vi "PS (single).vi"(8 "error in (no error)":errorcluster, 11 "XY-data":cluster{"X-array":dbl[], "Y-array":dbl[]} {"Y-array" format="%.2p"; "X-array" format="%.2p"}) -> (0 "error out":errorcluster, 2 "Power Spectrum":cluster{"f0":dbl, "df":dbl, "magnitude":dbl[]} {"magnitude" format="%.2p"; "f0" format="%0.2p"; "df" format="%0.2p"}, 3 "XY-data out":cluster{"X-array":dbl[], "Y-array":dbl[]} {"Y-array" format="%.2p"; "X-array" format="%.2p"})   [LabVIEW 2019, in "xy_utilities.lvlib"]
doc: "Computes the Power Spectrum of <B>XY-data</B>. This VI is a wrapper for NI_MAPro.lvlib:FFT Power Spectrum and PSD.vi.\n\nWire data to the data input to determine the polymorphic instance to use or manually select the instance."
uses:
  xy_utilities.lvlib
  <vilib>/measure/NI_MAPro.lvlib
  <vilib>/measure/maspectr.llb/FFT Power Spectrum and PSD for 1 Chan.vi
  <vilib>/measure/maspectr.llb/Power Spectrum and PSD Export Mode.ctl
  <vilib>/measure/maresamp.llb/Resample Pair of Arrays (single shot).vi
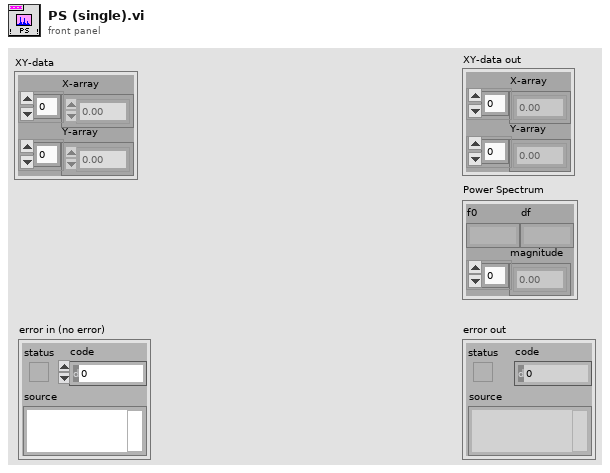
[diagram p1: front panel]
types:
  T1 = typedef "NI_MAPro.lvlib/Power Spectrum and PSD Export Mode.ctl" = u16
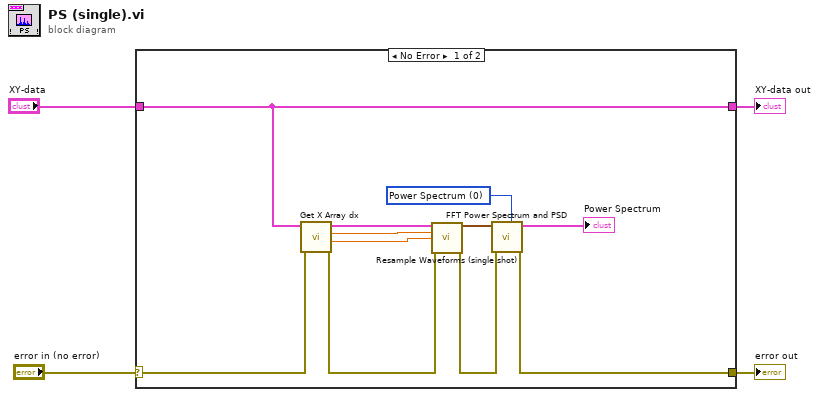
[diagram p0: block diagram]
diagram:
  n1 = case shown="No Error" "error in (no error)" {
    selector: "error in (no error)" -> [w6 w17]
    tunnel: [w12 w17] -> w3
    tunnel: "XY-data" -> [w5 w16]
    tunnel: [w5 w16] -> w1
    frame No Error {
      w11 = T1 0 items=["Power Spectrum", "Power Spectral Density"] ("export mode")
      n2 = call "Get X Array dx.vi"("error in (no error)"=w6, "XY-data"=w5) -> ("error out"=w7:errorcluster, "X0"=w8:dbl, "dX"=w9:dbl, "XY-data out"=w10:cluster{"X-array":dbl[], "Y-array":dbl[]})  [unwired: 6 in]
      n3 = call-poly <vilib>:"Resample Waveforms (single shot).vi"("XY-data in"=w10, "dt"=w9, "t0"=w8, "error in (no error)"=w7) -> ("resampled waveform out"=w15:waveform(dbl), "error out"=w13:errorcluster)  [unwired: 7 in, 3 out]
      n4 = call-poly <vilib>:"FFT Power Spectrum and PSD.vi"("export mode"=w11, "error in (no error)"=w13, "time signal"=w15) -> ("error out"=w12:errorcluster, "Power Spectrum / PSD"=→"Power Spectrum":cluster{"f0":dbl, "df":dbl, "magnitude":dbl[]})  [unwired: 5 in, 2 out]
    }
    frame Error {
    }
  }
  "error out" <- w3
  "XY-data out" <- w1
